vi "Path plus name.vi"(10 "Item Name":string, 11 "Object (or Item) Path":string) -> (1 "Number of Paths":i32, 2 "<JSON>End Name":string, 3 "Relative Path or JSON-format name":string)   [LabVIEW 2017, in "JSONtext.lvlib"]
uses:
  JSONtext.lvlib
  quote and escape json string 2.vi
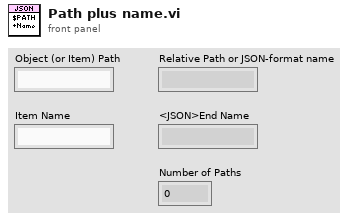
[diagram p1: front panel]
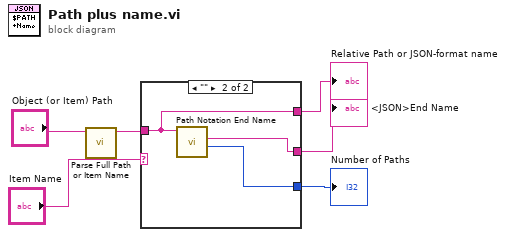
[diagram p0: block diagram]
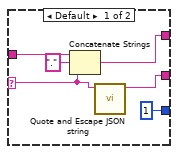
[diagram p2: hidden frame]
diagram:
  n1 = call "Parse Full Path or Item Name.vi"("Full Path (with $) or Name"="Object (or Item) Path") -> ("Relative Path or JSON-format name"=w6:string)  [unwired: 10 in]
  n2 = case shown="\"\"" "Item Name" {
    selector: "Item Name" -> [w8 _]
    tunnel: [w7 w14] -> w1
    tunnel: [1 w13] -> w2
    tunnel: w6 -> [w12 w15]
    tunnel: [w10 w15] -> w4
    frame Default {
      n3 = Concatenate Strings(w12, "." ("string"), w8) -> (w10:string)
      n4 = call "Quote and Escape JSON string.vi"("Plain Text"=w8) -> ("<JSON>"=w7:string)  [unwired: 10 in]
    }
    frame "" {
      n5 = call "Path Notation End Name.vi"("Item Path"=w15) -> ("Number of Paths"=w13:i32, "<JSON>End Name"=w14:string)  [unwired: 9 in]
    }
  }
  "Relative Path or JSON-format name" <- w4
  "Number of Paths" <- w2
  "<JSON>End Name" <- w1
